vi "SVI_SendSerialCommand.vi"(7 "Poll Time (ms)":u32=20, 8 "error in (no error)":errorcluster={"status"=FALSE, "code"=1073676294, "source"="VISA Read in SVI_ReadFromArduino.vi->FGV_SerialControl.vi"}, 9 "Voltage":dbl=704.0, 10 "Channel":u8, 11 "VISA Refnum in":refnum<visa-resource-name>="COM6") -> (0 "error out":errorcluster, 3 "VISA Refnum out":refnum<visa-resource-name>)   [LabVIEW 2020]
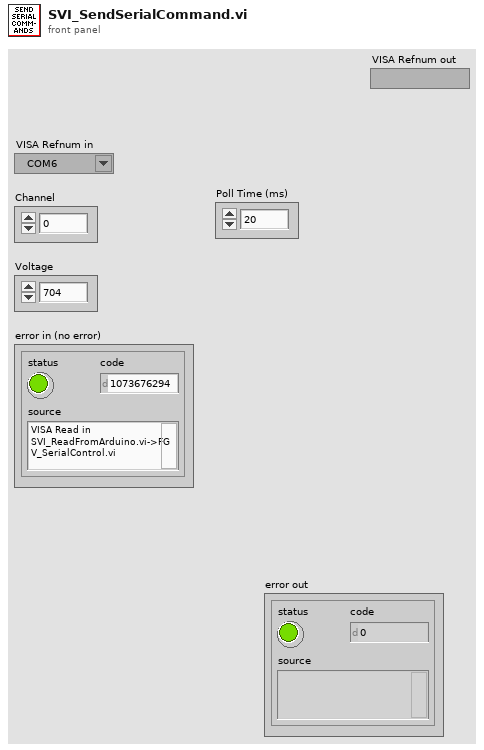
[diagram p1: front panel]
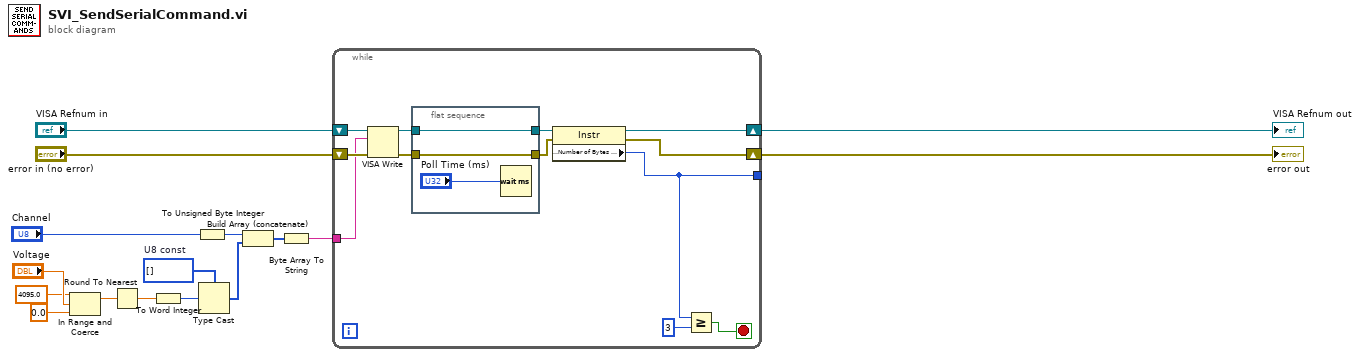
[diagram p0: block diagram]
diagram:
  w5 = u8[] []  # U8 const
  n1 = In Range and Coerce(upper limit=4095.0, x="Voltage", lower limit=0.0) -> (coerced(x)=w12:dbl)  [unwired: 1 out]
  n2 = Round To Nearest(number=w12) -> (nearest integer value=w8:dbl)
  n3 = To Word Integer(number=w8) -> (16bit integer=w7:i16)
  n4 = To Unsigned Byte Integer(number="Channel") -> (unsigned 8bit integer=w9:u8)
  n5 = Type Cast(type=w5, x=w7) -> (*(type *) &x=w6:u8[])
  n6 = Build Array (concatenate)(w9, w6) -> (w4:u8[])
  n7 = Byte Array To String(unsigned byte array=w4) -> (string=w3:string)
  n8 = while {
    tunnel: w3 -> [w26]
    tunnel: [w17] -> _
    shift-right: [w22] -> w1
    shift-left: "VISA Refnum in" -> [w28]
    shift-right: [w23] -> w2
    shift-left: "error in (no error)" -> [w27]
    stop <- w19 stop-if-true
    n9 = VISA Write(VISA resource name=w28, write buffer=w26, error in (no error)=w27) -> (VISA resource name out=w25:refnum<visa-resource-name>, error out=w24:errorcluster)  [unwired: 1 out]
    n10 = flat-sequence {
      tunnel: [w30] -> w20
      tunnel: w24 -> [w30]
      tunnel: [w29] -> w21
      tunnel: w25 -> [w29]
      frame #0 {
        n11 = Wait (ms)(milliseconds to wait="Poll Time (ms)") -> ()  [unwired: 1 out]
      }
    }
    n12 = property class="Instr"(reference=w21, error in=w20) -> (reference out=w22:refnum<visa-resource-name>, error out=w23:errorcluster, "Serial Settings:Number of Bytes at Serial Port"=w17:u32)
    n13 = Greater Or Equal?(x=w17, y=u32 3) -> (x >= y?=w19:bool)
  }
  "error out" <- w2
  "VISA Refnum out" <- w1
